vi "ARCO Main Server.vi"() -> ()   [LabVIEW 2017]
uses:
  <vilib>/OPCUA/controls/Data Type.ctl
  <vilib>/OPCUA/controls/Supported Security Policies.ctl
  <vilib>/OPCUA/NI OPC UA Server.lvlib
  <vilib>/OPCUA/NI OPC UA Utility.lvlib
panel:
  out "Result Boolean Control Node":string
  out "Result Numeric Control Node":string
  out "Result Data Node":string
  out "Spoof Boolean Control Node":string
  out "Spoof Numeric Control Node":string
  out "Spoof Data Node":string
  out "Chat Node":string
  out "Boolean Control Action Node":string
  out "Numeric Control Action Node":string
  out "certificate path 2":path
  out "certificate path":path
  out "error out":errorcluster
  out "CIET Data Node":string
  out "server endpoint URL":string
  in  "stop":bool
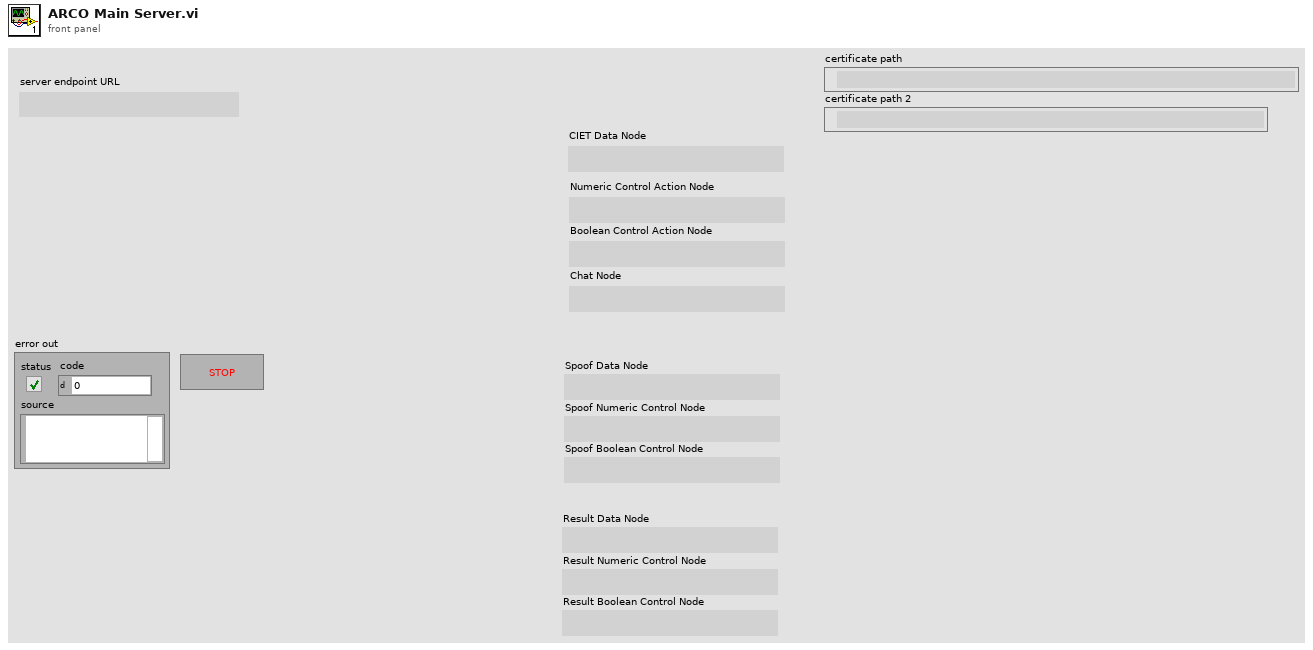
[diagram p1: front panel]
types:
  T1 = typedef "Data Type.ctl" = u16
  T2 = cluster{"name":string, "data type":T1, "access level":u16, "description":string}
  T3 = cluster{"name":string, "data type":T1, "access level 2":u16, "description":string}
  T4 = typedef "Supported Security Policies.ctl" = cluster{"None":bool, "Sign with Basic128Rsa15":bool, "Sign and Encrypt with Basic128Rsa15":bool, "Sign with Basic256":bool, "Sign and Encrypt with Basic256":bool}
  T5 = typedef "OPC UA Server Refnum.ctl" = refnum<k21>
  T6 = typedef "NodeId.ctl" = string
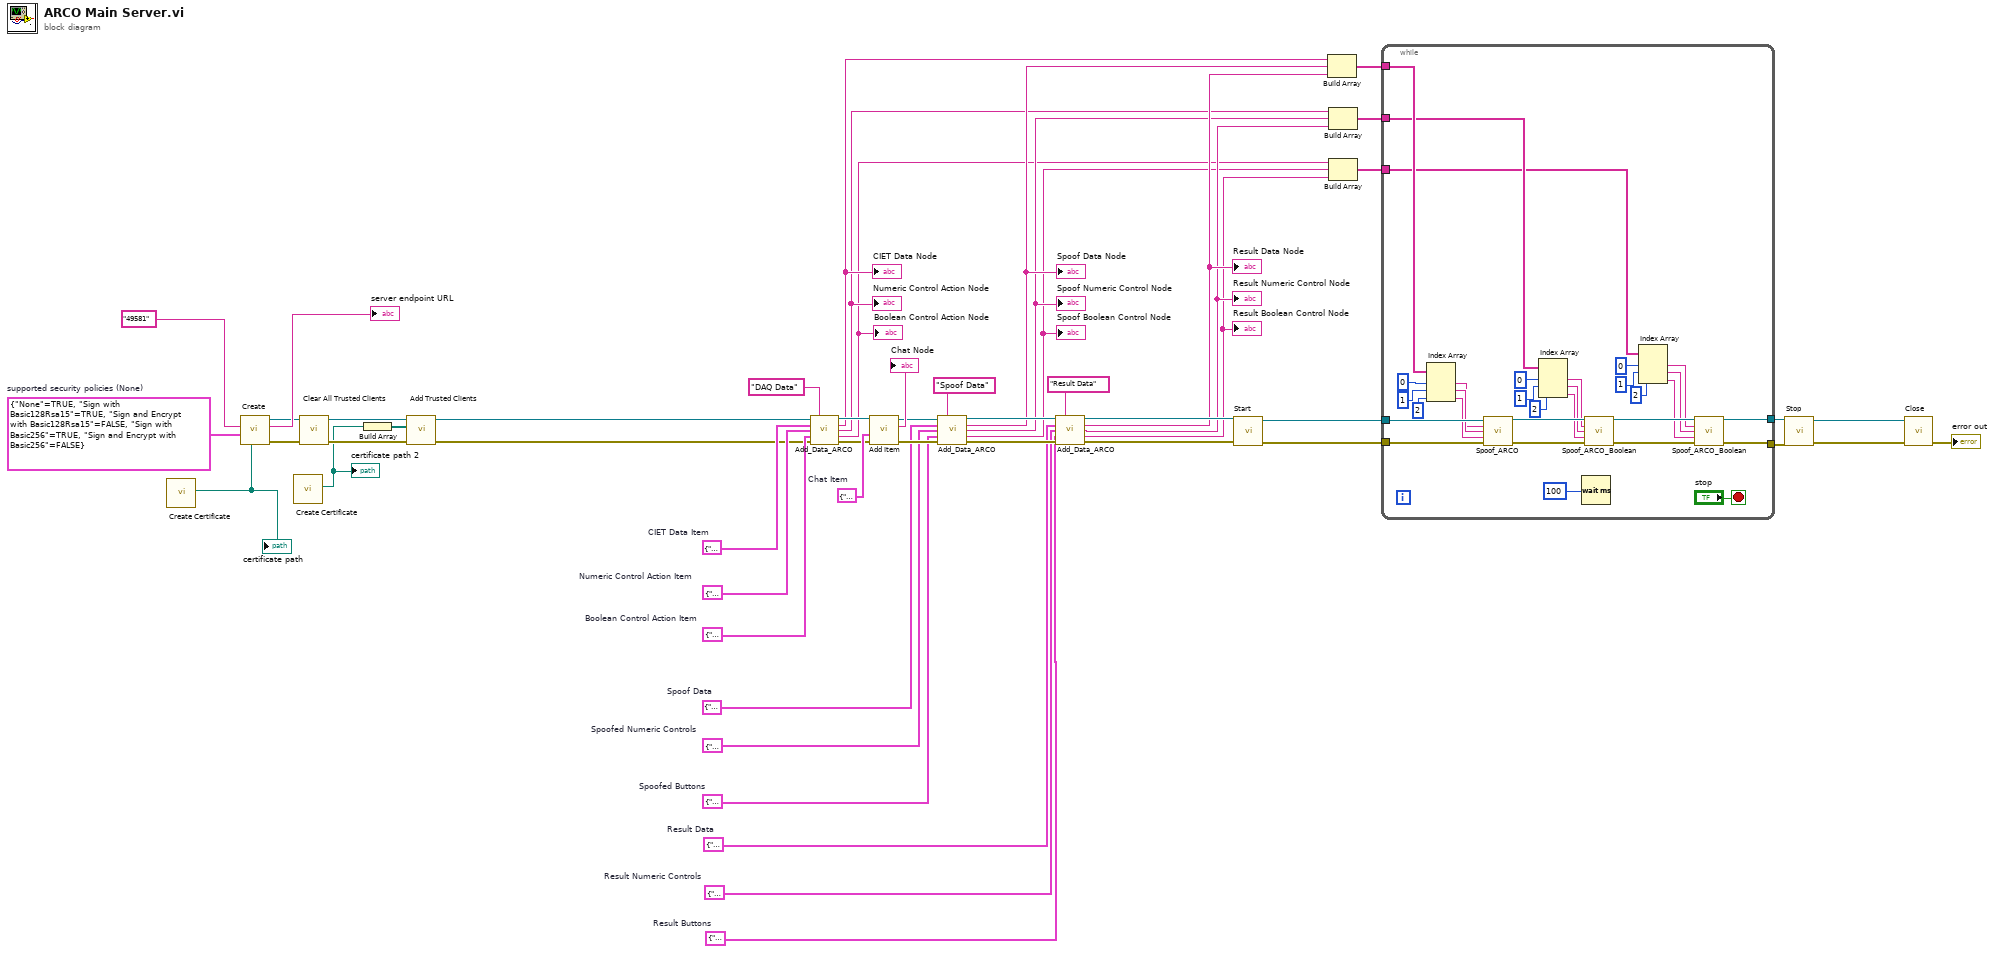
[diagram p0: block diagram]
diagram:
  w14 = T2 {"name"="Spoofed Numeric Controls", "data type"=111, "access level"=3, "description"="Spoofed Setpoints"}  # Spoofed Numeric Controls
  w15 = T2 {"name"="Spoofed CIET Data", "data type"=111, "access level"=3, "description"="Spoofed CIET TC and FM"}  # Spoof Data
  w22 = T2 {"name"="Result Boolean Controls", "data type"=101, "access level"=3, "description"="Result Buttons"}  # Result Buttons
  w23 = T2 {"name"="Result Numeric Controls", "data type"=111, "access level"=3, "description"="Result Setpoints"}  # Result Numeric Controls
  w24 = T3 {"name"="Result CIET Data", "data type"=111, "access level 2"=3, "description"="Result CIET TC and FM"}  # Result Data
  w13 = T2 {"name"="Spoofed Boolean Controls", "data type"=101, "access level"=3, "description"="Spoofed Buttons"}  # Spoofed Buttons
  w36 = T2 {"name"="Chat", "data type"=12, "access level"=3, "description"="Chat"}  # Chat Item
  w32 = T2 {"name"="Boolean Control Actions", "data type"=101, "access level"=3, "description"="Buttons"}  # Boolean Control Action Item
  w33 = T2 {"name"="Numeric Control Actions", "data type"=111, "access level"=3, "description"="Setpoints"}  # Numeric Control Action Item
  w45 = T4 {"None"=TRUE, "Sign with Basic128Rsa15"=TRUE, "Sign and Encrypt with Basic128Rsa15"=FALSE, "Sign with Basic256"=TRUE, "Sign and Encrypt with Basic256"=FALSE}  # supported security policies (None)
  w34 = T2 {"name"="CIET Data", "data type"=111, "access level"=3, "description"="CIET TC and FM"}  # CIET Data Item
  n1 = call <vilib>:"Create Certificate.vi"() -> ("certificate path"=w40:path)  [unwired: 8 in, 3 out]
  "certificate path" <- w40
  n2 = call <vilib>:"Create.vi"("server certificate file"=w40, "supported security policies (None)"=w45, "TCP port (49580)"="49581") -> ("error out"=w41:errorcluster, "server endpoint URL"=→"server endpoint URL":string, "OPC UA server refnum out"=w42:T5)  [unwired: 6 in]
  n3 = call <vilib>:"Create Certificate.vi"() -> ("certificate path"=w39:path)  [unwired: 8 in, 3 out]
  "certificate path 2" <- w39
  n4 = call <vilib>:"Clear All Trusted Clients.vi"("error in (no error)"=w41, "OPC UA server refnum in"=w42) -> ("error out"=w43:errorcluster, "OPC UA server refnum out"=w44:T5)  [unwired: 8 in]
  n5 = Build Array(w39) -> (w38:path[])
  n6 = call <vilib>:"Add Trusted Clients.vi"("error in (no error)"=w43, "trusted client certificates"=w38, "OPC UA server refnum in"=w44) -> ("error out"=w16:errorcluster, "OPC UA server refnum out"=w17:T5)  [unwired: 7 in]
  n7 = call "Add_Data_ARCO.vi"("Refnum in"=w17, "folder name"="DAQ Data", "item 1"=w34, "item 2"=w33, "item 3"=w32, "error in (no error)"=w16) -> ("Refnum out"=w31:T5, "item node ID 1"=w9:string, "item node ID 2"=w6:string, "item node ID 3"=w3:string, "error out"=w30:errorcluster)  [unwired: 5 in]
  "CIET Data Node" <- w9
  "Numeric Control Action Node" <- w6
  "Boolean Control Action Node" <- w3
  n8 = call <vilib>:"Add Item.vi"("error in (no error)"=w30, "item"=w36, "OPC UA server refnum in"=w31) -> ("error out"=w27:errorcluster, "item node ID"=→"Chat Node":T6, "OPC UA server refnum out"=w28:T5)  [unwired: 4 in, 1 out]
  n9 = call "Add_Data_ARCO.vi"("Refnum in"=w28, "folder name"="Spoof Data", "item 1"=w15, "item 2"=w14, "item 3"=w13, "error in (no error)"=w27) -> ("Refnum out"=w25:T5, "item node ID 1"=w8:string, "item node ID 2"=w5:string, "item node ID 3"=w2:string, "error out"=w26:errorcluster)  [unwired: 5 in]
  "Spoof Data Node" <- w8
  "Spoof Numeric Control Node" <- w5
  "Spoof Boolean Control Node" <- w2
  n10 = call "Add_Data_ARCO.vi"("Refnum in"=w25, "folder name"="Result Data", "item 1"=w24, "item 2"=w23, "item 3"=w22, "error in (no error)"=w26) -> ("Refnum out"=w18:T5, "item node ID 1"=w7:string, "item node ID 2"=w4:string, "item node ID 3"=w1:string, "error out"=w19:errorcluster)  [unwired: 5 in]
  "Result Data Node" <- w7
  "Result Numeric Control Node" <- w4
  "Result Boolean Control Node" <- w1
  n11 = call <vilib>:"Start.vi"("error in (no error)"=w19, "OPC UA server refnum in"=w18) -> ("error out"=w51:errorcluster, "OPC UA server refnum out"=w52:T5)  [unwired: 7 in, 1 out]
  n12 = Build Array(w9, w8, w7) -> (w12:string[])
  n13 = Build Array(w6, w5, w4) -> (w11:string[])
  n14 = Build Array(w3, w2, w1) -> (w10:string[])
  n15 = while {
    tunnel: [w80] -> w49
    tunnel: w52 -> [w75]
    tunnel: [w79] -> w50
    tunnel: w51 -> [w78]
    tunnel: w12 -> [w56]
    tunnel: w11 -> [w55]
    tunnel: w10 -> [w54]
    stop <- "stop" stop-if-true
    n16 = Index Array(array=w56, index #1=0, index #2=1, index #3=2) -> (element #1=w69:string, element #2=w70:string, element #3=w71:string)
    n17 = call "Spoof_ARCO.vi"("OPC UA server refnum in"=w75, "DAQ Node"=w69, "Spoof Node"=w70, "Result Node"=w71, "error in (no error)"=w78) -> ("OPC UA server refnum out"=w76:T5, "error out"=w77:errorcluster)  [unwired: 9 in]
    n18 = Index Array(array=w55, index #1=0, index #2=1, index #3=2) -> (element #1=w63:string, element #2=w64:string, element #3=w65:string)
    n19 = Wait (ms)(milliseconds to wait=u32 100) -> ()  [unwired: 1 out]
    n20 = call "Spoof_ARCO_Boolean.vi"("OPC UA server refnum in"=w76, "Spoof Node"=w63, "DAQ Node"=w64, "Result Node"=w65, "error in (no error)"=w77) -> ("OPC UA server refnum out"=w82:T5, "error out"=w81:errorcluster)  [unwired: 9 in]
    n21 = Index Array(array=w54, index #1=0, index #2=1, index #3=2) -> (element #1=w57:string, element #2=w58:string, element #3=w59:string)
    n22 = call "Spoof_ARCO_Boolean.vi"("OPC UA server refnum in"=w82, "Spoof Node"=w57, "DAQ Node"=w58, "Result Node"=w59, "error in (no error)"=w81) -> ("OPC UA server refnum out"=w80:T5, "error out"=w79:errorcluster)  [unwired: 9 in]
  }
  n23 = call <vilib>:"Stop.vi"("error in (no error)"=w50, "OPC UA server refnum in"=w49) -> ("error out"=w47:errorcluster, "OPC UA server refnum out"=w48:T5)  [unwired: 8 in]
  n24 = call <vilib>:"Close.vi"("error in (no error)"=w47, "OPC UA server refnum in"=w48) -> ("error out"=→"error out":errorcluster)  [unwired: 9 in]
